vi "Log 2D Table.vi"(0 "Log Path":path, 2 "Replace File":bool, 7 "Table Data IN":string[][](array[string]), 11 "Error IN":errorcluster) -> (15 "Error OUT":errorcluster)   [LabVIEW 2011]
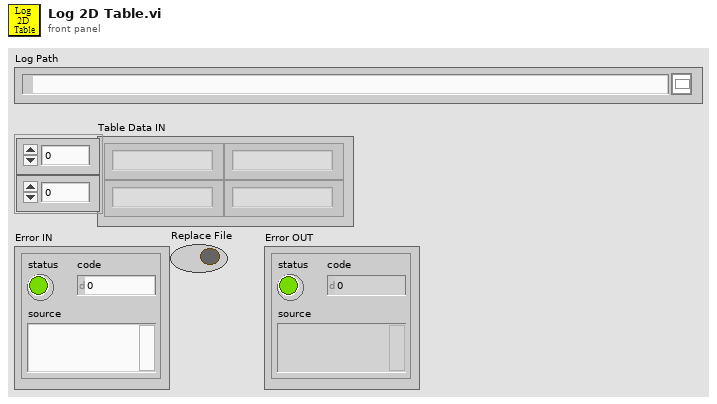
[diagram p1: front panel]
types:
  T1 = enum16{"open", "replace", "create", "open or create", "replace or create", "replace or create with confirmation"}
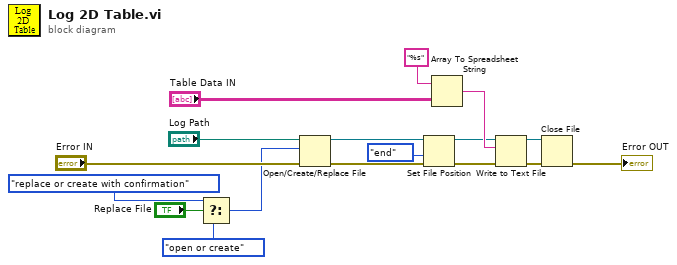
[diagram p0: block diagram]
diagram:
  n1 = Select(t=T1."replace or create with confirmation" ("operation (0:open)"), s="Replace File", f=T1."open or create" ("operation (0:open)")) -> (s? t:f=w1:T1)
  n2 = Open/Create/Replace File(file path (use dialog)="Log Path", error in="Error IN", operation (0:open)=w1) -> (refnum out=w9:refnum<file>, error out=w8:errorcluster)  [unwired: 3 in, 1 out]
  n3 = Set File Position(refnum=w9, from (0:start)=enum16{"start", "end", "current"}."end", error in=w8) -> (refnum out=w10:refnum<file>, error out=w7:errorcluster)  [unwired: 1 in]
  n4 = Array To Spreadsheet String(array="Table Data IN", 3:"%s" ("format (%s)")) -> (spreadsheet string=w13:string)  [unwired: 1 in]
  n5 = Write to Text File(file (use dialog)=w10, text=w13, error in=w7) -> (refnum out=w5:refnum<file>, error out=w6:errorcluster)  [unwired: 1 in, 1 out]
  n6 = Close File(refnum=w5, error in=w6) -> (error out=→"Error OUT":errorcluster)  [unwired: 1 out]
